vi "I2C_GetRawAcceleration.vi"(11 "navX DevRef":T1={"I2CDevRef"={"DevStatus"={"status"=FALSE, "code"=0, "source"=""}, "Controller"=enum."Controller 1", "Device Address"=0, "Handle"=0, "I2C Bus"=enum."Invalid"}, "Board Information"={"WhoAmI (50 | 0x32)"=0, "Board Revision"=0, "Firmware Major Version"=0, "Firmware Minor Version"=0}, "Status"={"Update Rate Hz"=0, "Accelerometer Full-Scale Range"=0, "Gyro Full-Scale Range"=0, "NAVX_OP_STATUS"=0, "NAVX_CAL_STATUS"=0, "NAVX_SELFTEST_STATUS"=0, "NAVX_SENSOR_STATUS"={"MOVING"=FALSE, "YAW_STABLE"=FALSE, "MAG_DISTURBANCE"=FALSE, "ALTITUDE_VALID"=FALSE, "SEALEVEL_PRESS_SET"=FALSE, "FUSED_HEADING_VALID"=FALSE}}, "Offsets"={"Yaw"=0.0, "Quat W"=0.0, "Quat X"=0.0, "Quat Y"=0.0, "Quat Z"=0.0}, "Update Rate (4Hz-60Hz)"=50, "refnum name"="", "error"={"status"=FALSE, "code"=0, "source"=""}} {"I2CDevRef"."Device Address" format="%.0x"; "Status"."NAVX_OP_STATUS" items=["INITIALIZING", "SELFTEST_IN_PROGRESS", "ERROR", "IMU_AUTOCAL_IN_PROGRESS", "NORMAL"]; "Status"."NAVX_CAL_STATUS" items=["IMU_CAL_STATE_MASK"=3, "IMU_CAL_INPROGRESS"=0, "IMU_CAL_ACCUMULATE"=1, "IMU_CAL_COMPLETE"=2, "MAG_CAL_COMPLETE"=4, "BARO_CAL_COMPLETE"=8]}) -> (2 "Vector":T10, 3 "navX DevRef":T1={"I2CDevRef"={"DevStatus"={"status"=FALSE, "code"=0, "source"=""}, "Controller"=enum."Controller 1", "Device Address"=0, "Handle"=0, "I2C Bus"=enum."Invalid"}, "Board Information"={"WhoAmI (50 | 0x32)"=0, "Board Revision"=0, "Firmware Major Version"=0, "Firmware Minor Version"=0}, "Status"={"Update Rate Hz"=0, "Accelerometer Full-Scale Range"=0, "Gyro Full-Scale Range"=0, "NAVX_OP_STATUS"=0, "NAVX_CAL_STATUS"=0, "NAVX_SELFTEST_STATUS"=0, "NAVX_SENSOR_STATUS"={"MOVING"=FALSE, "YAW_STABLE"=FALSE, "MAG_DISTURBANCE"=FALSE, "ALTITUDE_VALID"=FALSE, "SEALEVEL_PRESS_SET"=FALSE, "FUSED_HEADING_VALID"=FALSE}}, "Offsets"={"Yaw"=0.0, "Quat W"=0.0, "Quat X"=0.0, "Quat Y"=0.0, "Quat Z"=0.0}, "Update Rate (4Hz-60Hz)"=50, "refnum name"="", "error"={"status"=FALSE, "code"=0, "source"=""}} {"I2CDevRef"."Device Address" format="%.0x"; "Status"."NAVX_OP_STATUS" items=["INITIALIZING", "SELFTEST_IN_PROGRESS", "ERROR", "IMU_AUTOCAL_IN_PROGRESS", "NORMAL"]; "Status"."NAVX_CAL_STATUS" items=["IMU_CAL_STATE_MASK"=3, "IMU_CAL_INPROGRESS"=0, "IMU_CAL_ACCUMULATE"=1, "IMU_CAL_COMPLETE"=2, "MAG_CAL_COMPLETE"=4, "BARO_CAL_COMPLETE"=8]})   [LabVIEW 2014, in "navX-MXP IMU.lvlib"]
uses:
  navX-MXP IMU.lvlib
  TypeDefs/navX I2C DevRef.ctl
  <vilib>/Rock Robotics/WPI/I2C/WPI_I2CDevRef.ctl
  <vilib>/Rock Robotics/SystemInterfaces/Typedef/FPGA_TypedefDigitalModule.ctl
  <vilib>/Rock Robotics/SystemInterfaces/i2clib/i2c_bus.ctl
  COMMON/TypeDefs/Data TypeDefs/navX Board Information.ctl
  COMMON/TypeDefs/Data TypeDefs/navX Status Data.ctl
  COMMON/TypeDefs/Value TypeDefs/navX NAVX_OP_STATUS.ctl
  COMMON/TypeDefs/Value TypeDefs/navX NAVX_CAL_STATUS.ctl
  COMMON/TypeDefs/Value TypeDefs/navX NAVX_SENSOR_STATUS.ctl
  COMMON/TypeDefs/Data TypeDefs/navX Vector Data.ctl
  COMMON/TypeDefs/Value TypeDefs/navX Device Registers.ctl
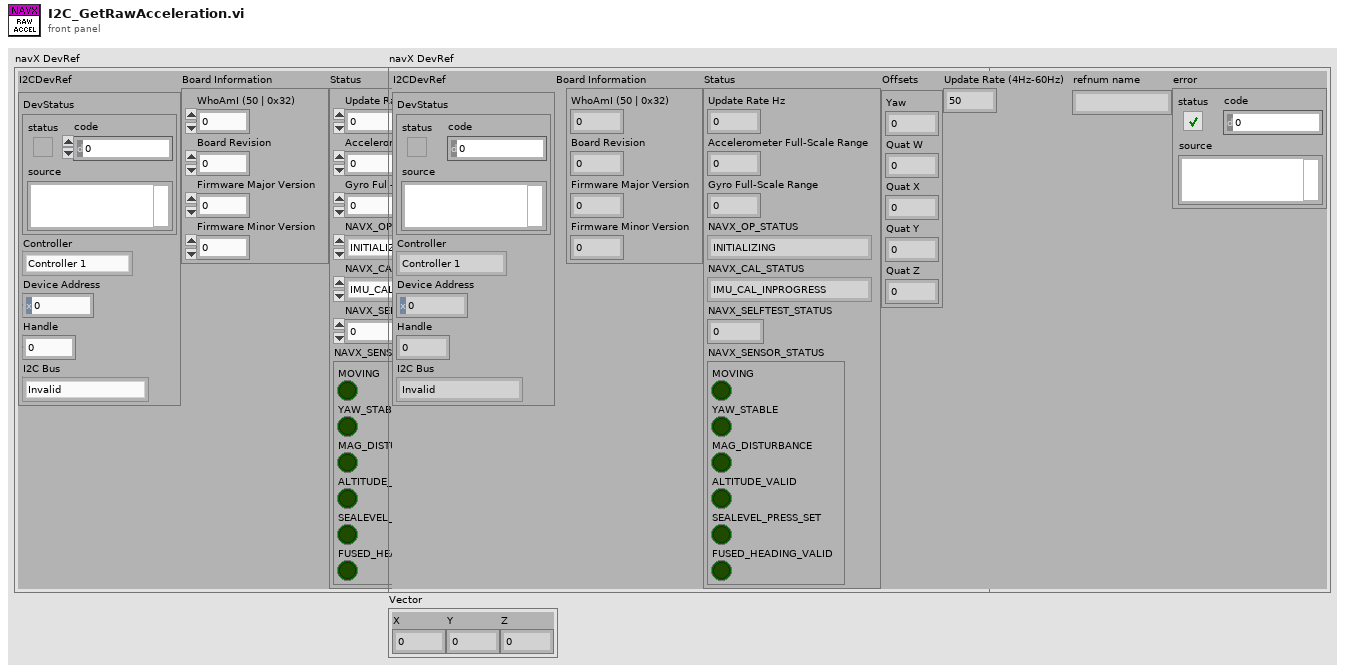
[diagram p1: front panel]
types:
  T1 = typedef "navX-MXP IMU.lvlib/navX I2C DevRef.ctl" = cluster{"I2CDevRef":T2, "Board Information":T5, "Status":T6, "Offsets":cluster{"Yaw":dbl, "Quat W":dbl, "Quat X":dbl, "Quat Y":dbl, "Quat Z":dbl}, "Update Rate (4Hz-60Hz)":u8, "refnum name":string, "error":errorcluster}
  T2 = typedef "WPI_I2CDevRef.ctl" = cluster{"DevStatus":errorcluster, "Controller":T3, "Device Address":u8, "Handle":i32, "I2C Bus":T4}
  T3 = typedef "FPGA_TypedefDigitalModule.ctl" = enum16{"Controller 1"}
  T4 = typedef "i2c_bus.ctl" = enum16{"I2C On-Board", "I2C MXP", "Invalid"}
  T5 = typedef "navX-MXP IMU.lvlib/navX Board Information.ctl" = cluster{"WhoAmI (50 | 0x32)":u8, "Board Revision":u8, "Firmware Major Version":u8, "Firmware Minor Version":u8}
  T6 = typedef "navX-MXP IMU.lvlib/navX Status Data.ctl" = cluster{"Update Rate Hz":u8, "Accelerometer Full-Scale Range":u8, "Gyro Full-Scale Range":u16, "NAVX_OP_STATUS":T7, "NAVX_CAL_STATUS":T8, "NAVX_SELFTEST_STATUS":u8, "NAVX_SENSOR_STATUS":T9}
  T7 = typedef "navX-MXP IMU.lvlib/navX NAVX_OP_STATUS.ctl" = u8
  T8 = typedef "navX-MXP IMU.lvlib/navX NAVX_CAL_STATUS.ctl" = u8
  T9 = typedef "navX-MXP IMU.lvlib/navX NAVX_SENSOR_STATUS.ctl" = cluster{"MOVING":bool, "YAW_STABLE":bool, "MAG_DISTURBANCE":bool, "ALTITUDE_VALID":bool, "SEALEVEL_PRESS_SET":bool, "FUSED_HEADING_VALID":bool}
  T10 = typedef "navX-MXP IMU.lvlib/navX Vector Data.ctl" = cluster{"X":dbl, "Y":dbl, "Z":dbl}
  T11 = typedef "navX-MXP IMU.lvlib/navX Device Registers.ctl" = u8
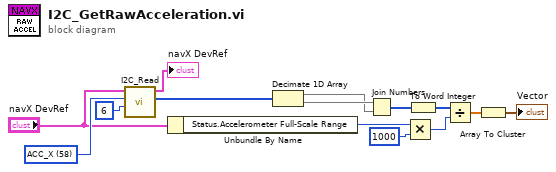
[diagram p0: block diagram]
diagram:
  w14 = T11 58 items=["WHOAMI"=0, "HW_REV"=1, "FW_VER_MAJOR"=2, "FW_VER_MINOR"=3, "UPDATE_RATE_HZ"=4, "ACCEL_FSR_G"=5, "GYRO_FSR_DPS"=6, "OP_STATUS"=8, "CAL_STATUS"=9, "SELFTEST_STATUS"=10, "SENSOR_STATUS"=16, "TIMESTAMP"=18, "YAW"=22, "PITCH"=24, "ROLL"=26, "HEADING"=28, "FUSED_HEADING"=30, "ALTITUDE_I"=32, "ALTITUDE_D"=34, "LINERA_ACC_X"=36, "LINERA_ACC_Y"=38, "LINERA_ACC_Z"=40, "QUAT_W"=42, "QUAT_X"=44, "QUAT_Y"=46, "QUAT_Z"=48, "MPU_TEMP_C"=50, "GYRO_X"=52, "GYRO_Y"=54, "GYRO_Z"=56, "ACC_X"=58, "ACC_Y"=60, "ACC_Z"=62, "MAG_X"=64, "MAG_Y"=66, "MAG_Z"=68, "PRESSURE_I"=70, "PRESSURE_D"=72, "PRESSURE_TEMP"=74, "YAW_OFFSET"=76, "QUAT_OFFSET_W"=78, "QUAT_OFFSET_X"=80, "QUAT_OFFSET_Y"=82, "QUAT_OFFSET_Z"=84] ("Device Register")
  n1 = call "I2C_Read.vi"("Read Size"=u8 6 ("Data To Send"), "Device Register"=w14, "navX DevRef"="navX DevRef") -> ("navX Data"=w5:u8[], "navX DevRef"=→"navX DevRef":T1)  [unwired: 7 in]
  n2 = Unbundle By Name("navX DevRef") -> ("Status.Accelerometer Full-Scale Range"=w12:u8)
  n3 = Decimate 1D Array(w5) -> (w9:u8[], w10:u8[])
  n4 = Join Numbers(hi=w10, lo=w9) -> ((hi.lo)=w8:u16[])
  n5 = Multiply(x=w12, y=u16 1000) -> (x*y=w3:u16)
  n6 = To Word Integer(number=w8) -> (16bit integer=w7:i16[])
  n7 = Divide(x=w7, y=w3) -> (x/y=w6:dbl[])
  n8 = Array To Cluster(array=w6) -> (cluster=→"Vector":cluster{"[0]":dbl, "[1]":dbl, "[2]":dbl})
